vi "setOptions.vi"(8 "error in (no error)":errorcluster, 10 "Options":T1, 11 "tBSONRegEx in":refnum<class "tBSONRegEx.lvclass">) -> (0 "error out":errorcluster, 3 "tBSONRegEx out":refnum<class "tBSONRegEx.lvclass">)   [LabVIEW 2013, in "BSON.lvlib" / "tBSONRegEx.lvclass"]
uses:
  tBSONRegEx.lvclass
  options.ctl
  tBSONRegEx.lvclass/tBSONRegEx.ctl
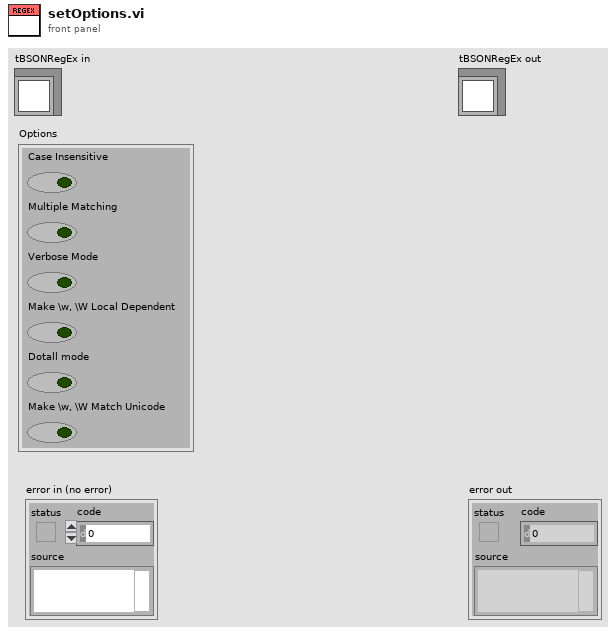
[diagram p1: front panel]
types:
  T1 = typedef "BSON.lvlib/tBSONRegEx.lvclass/options.ctl" = cluster{"Case Insensitive":bool, "Multiple Matching":bool, "Verbose Mode":bool, "Make \\w, \\W Local Dependent":bool, "Dotall mode":bool, "Make \\w, \\W Match Unicode":bool}
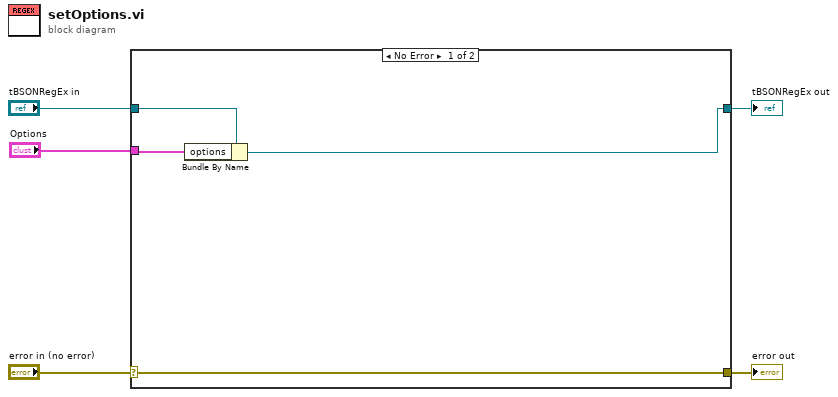
[diagram p0: block diagram]
diagram:
  n1 = case shown="No Error" "error in (no error)" {
    selector: "error in (no error)" -> [w9 w11]
    tunnel: [w9 w11] -> w4
    tunnel: [w6 w10] -> w2
    tunnel: "tBSONRegEx in" -> [w7 w10]
    tunnel: "Options" -> [w8 _]
    frame No Error {
      n2 = Bundle By Name(cluster=w7, "options"=w8) -> (w6:refnum<class "tBSONRegEx.lvclass">)
    }
    frame Error {
    }
  }
  "error out" <- w4
  "tBSONRegEx out" <- w2
